vi "FL Create Rule.vi"(4 "consequent implication":T6 items=["Minimum", "Product"], 5 "antecedent connective":T4 items=["AND (Minimum)", "AND (Product)", "OR (Maximum)", "OR (Probabilistic)"], 6 "consequents":T5[](array[typedef]) {"Var Index" min=0; "Cond" items=["=", "!="]; "MF Index" min=0}, 7 "antecedents":T2[](array[typedef]) {"Var Index" min=0; "Cond" items=["=", "!="]; "MF Index" min=0}, 8 "error in (no error)":errorcluster, 9 "degree of support (1)":dbl=1.0) -> (0 "error out":errorcluster, 3 "rule":T1={"antecedents"=[], "antecedent connective"=0, "consequents"=[], "consequent implication"=0, "degree of support"=1.0} {"consequents"."Var Index" min=0; "consequents"."Cond" items=["=", "!="]; "consequents"."MF Index" min=0; "antecedents"."Var Index" min=0; "antecedents"."Cond" items=["=", "!="]; "antecedents"."MF Index" min=0; "consequent implication" items=["Minimum", "Product"]; "antecedent connective" items=["AND (Minimum)", "AND (Product)", "OR (Maximum)", "OR (Probabilistic)"]})   [LabVIEW 2017, in "NI_Fuzzy_Logic_API.lvlib"]
doc: "Creates a rule for a fuzzy system. You also can use the <B>Rule Editor</B> page of the Fuzzy System Designer to create rules interactively."
uses:
  <vilib>/addons/Fuzzy Logic/NI_Fuzzy_Logic_API.lvlib
  <vilib>/addons/Fuzzy Logic/TypeDefs/FL Antecedent.ctl
  <vilib>/addons/Fuzzy Logic/TypeDefs/FL Modifier.ctl
  <vilib>/addons/Fuzzy Logic/TypeDefs/FL Consequent.ctl
  <vilib>/addons/Fuzzy Logic/TypeDefs/FL Antecedent Connective.ctl
  <vilib>/addons/Fuzzy Logic/TypeDefs/FL Consequent Implication.ctl
  <vilib>/addons/Fuzzy Logic/TypeDefs/FL Rule.ctl
panel:
  # "IF"
  # "THEN"
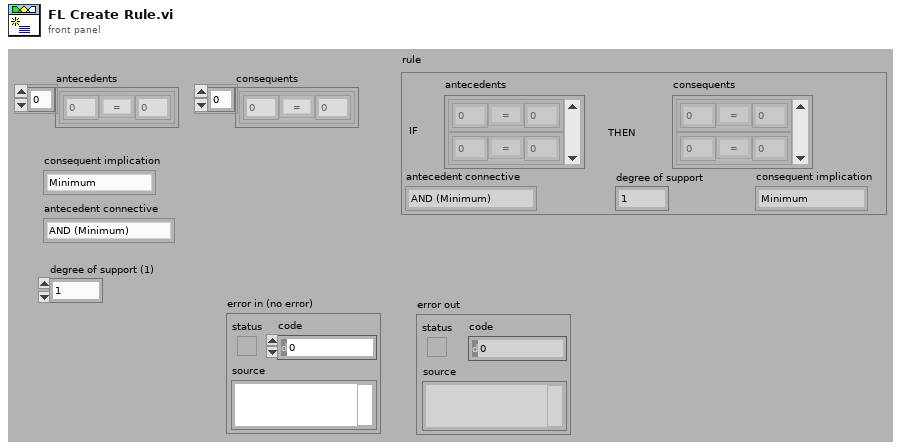
[diagram p1: front panel]
types:
  T1 = typedef "NI_Fuzzy_Logic_API.lvlib/FL Rule.ctl" = cluster{"antecedents":T2[], "antecedent connective":T4, "consequents":T5[], "consequent implication":T6, "degree of support":dbl}
  T2 = typedef "NI_Fuzzy_Logic_API.lvlib/FL Antecedent.ctl" = cluster{"Var Index":i32, "MF Index":i32, "Cond":T3}
  T3 = typedef "NI_Fuzzy_Logic_API.lvlib/FL Modifier.ctl" = u16
  T4 = typedef "NI_Fuzzy_Logic_API.lvlib/FL Antecedent Connective.ctl" = u16
  T5 = typedef "NI_Fuzzy_Logic_API.lvlib/FL Consequent.ctl" = cluster{"Var Index":i32, "MF Index":i32, "Cond":T3}
  T6 = typedef "NI_Fuzzy_Logic_API.lvlib/FL Consequent Implication.ctl" = u16
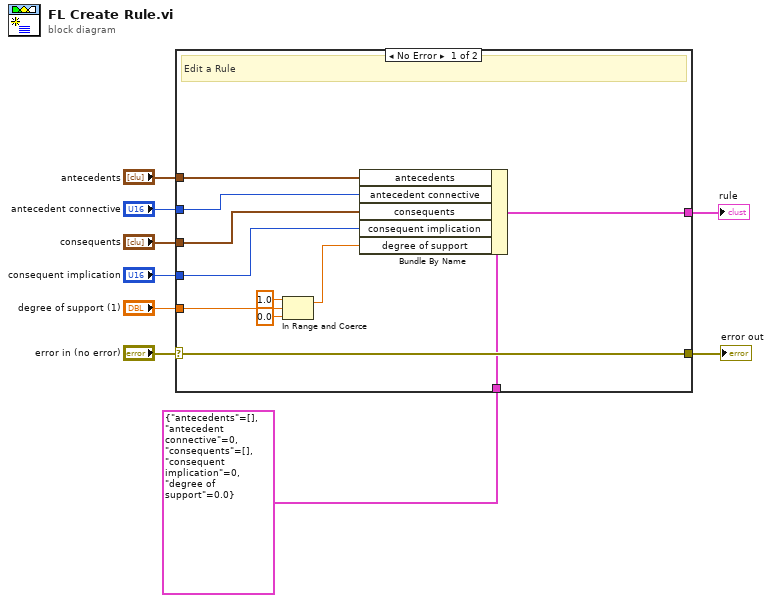
[diagram p0: block diagram]
diagram:
  n1 = case shown="No Error" "error in (no error)" {
    selector: "error in (no error)" -> [w17 w22]
    tunnel: "antecedents" -> [w16 _]
    tunnel: "antecedent connective" -> [w14 _]
    tunnel: "consequents" -> [w13 _]
    tunnel: "degree of support (1)" -> [w18 _]
    tunnel: "consequent implication" -> [w12 _]
    tunnel: [w17 w22] -> w3
    tunnel: [w15 w21] -> w2
    tunnel: T1 {"antecedents"=[], "antecedent connective"=0, "consequents"=[], "consequent implication"=0, "degree of support"=0.0} ("rule") -> [w10 w21]
    frame No Error {
      # "Edit a Rule"
      n2 = In Range and Coerce(upper limit=1.0, x=w18, lower limit=0.0) -> (coerced(x)=w11:dbl)  [unwired: 1 out]
      n3 = Bundle By Name(cluster=w10, "antecedents"=w16, "antecedent connective"=w14, "consequents"=w13, "consequent implication"=w12, "degree of support"=w11) -> (w15:T1)
    }
    frame Error {
    }
  }
  "error out" <- w3
  "rule" <- w2
